vi "Close.vi"(8 "error in (no error)":errorcluster, 11 "Abstract Message Queue in":refnum<class "Abstract Message Queue.lvclass">) -> (0 "error out":errorcluster, 3 "Abstract Message Queue out":refnum<class "Abstract Message Queue.lvclass">)   [LabVIEW 2017, in "Messaging.lvlib" / "Abstract Message Queue.lvclass"]
uses:
  Abstract Message Queue.lvclass
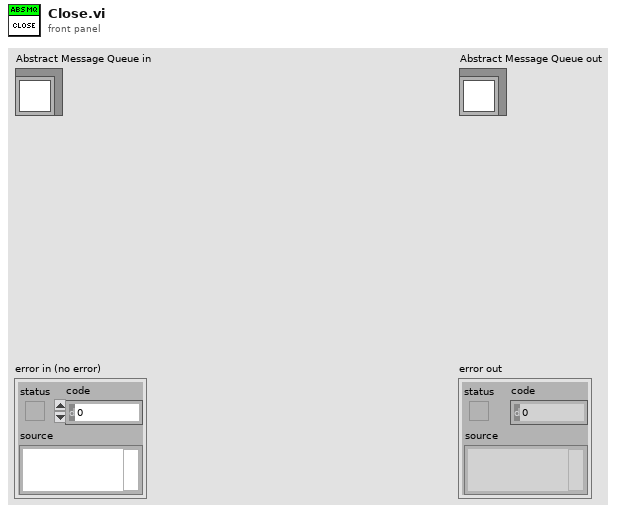
[diagram p1: front panel]
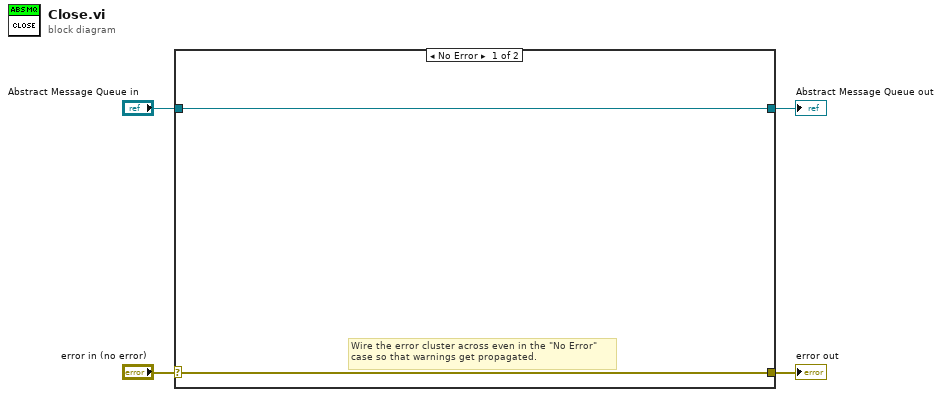
[diagram p0: block diagram]
diagram:
  n1 = case shown="No Error" "error in (no error)" {
    selector: "error in (no error)" -> [w5 w8]
    tunnel: [w5 w8] -> w3
    tunnel: [w6 w7] -> w1
    tunnel: "Abstract Message Queue in" -> [w6 w7]
    frame No Error {
      # "Wire the error cluster across even in the \"No Error\"\ncase so that warnings get propagated."
    }
    frame Error {
    }
  }
  "error out" <- w3
  "Abstract Message Queue out" <- w1
